vi "Linear Shifter.vi"(9 "Shift":dbl, 11 "Input":dbl) -> (3 "Output":dbl)   [LabVIEW 2012]
panel:
  out "mx+b":dbl
  out "m*x":dbl
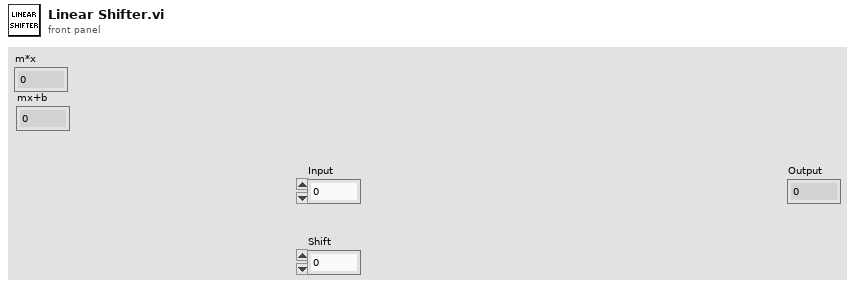
[diagram p1: front panel]
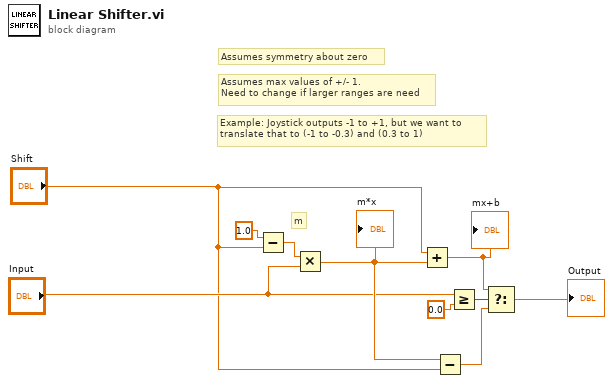
[diagram p0: block diagram]
diagram:
  # "Assumes max values of +/- 1.\nNeed to change if larger ranges are need"
  # "Assumes symmetry about zero"
  # "Example: Joystick outputs -1 to +1, but we want to\ntranslate that to (-1 to -0.3) and (0.3 to 1)"
  # "m"
  n1 = Subtract(x=1.0, y="Shift") -> (x-y=w7:dbl)
  n2 = Multiply(x=w7, y="Input") -> (x*y=w5:dbl)
  "m*x" <- w5
  n3 = Add(x="Shift", y=w5) -> (x+y=w6:dbl)
  "mx+b" <- w6
  n4 = Subtract(x=w5, y="Shift") -> (x-y=w4:dbl)
  n5 = Greater Or Equal?(x="Input", y=0.0) -> (x >= y?=w9:bool)
  n6 = Select(t=w6, s=w9, f=w4) -> (s? t:f=→"Output":dbl)
